vi "Timeseries 1D to XY.vi"(7 "Swap axes":bool, 11 "Waveform New":cluster{dbl, dbl, dbl[]}) -> (3 "output cluster":cluster{dbl[], dbl[]})   [LabVIEW 2016]
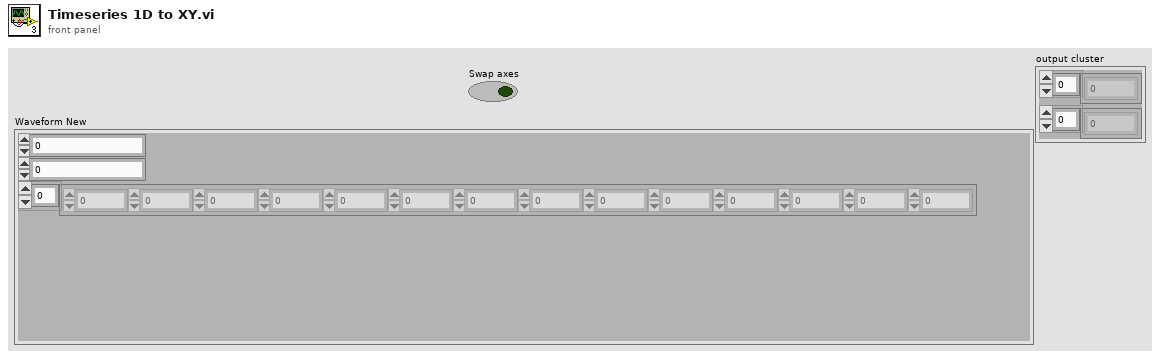
[diagram p1: front panel]
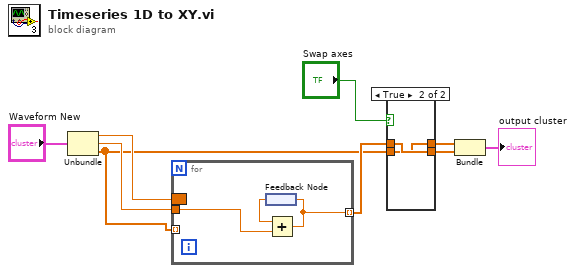
[diagram p0: block diagram]
diagram:
  n1 = Unbundle("Waveform New") -> (w7:dbl, w8:dbl, w3:dbl[])
  n2 = for {
    tunnel: w3 -> [_] mode=indexing
    tunnel: w8 -> [w12]
    border: w7 -> [_]
    tunnel: [w10] -> w4 mode=indexing
    n3 = feedback #1() -> (w11:dbl)
    n4 = Add(x=w11, y=w12) -> (x+y=w10:dbl)
    n5 = feedback-in #1(w10) -> ()
  }
  n6 = case shown="True" "Swap axes" {
    tunnel: w4 -> [w14 w16]
    tunnel: w3 -> [w13 w15]
    tunnel: [w14 w15] -> w2
    tunnel: [w13 w16] -> w1
    frame False {
    }
    frame True {
    }
  }
  n7 = Bundle(w2, w1) -> (→"output cluster":cluster{dbl[], dbl[]})  [unwired: 1 in]
